vi "InitializeFunctionList.vi"(8 "错误输入（无错误）":errorcluster, 9 "模块定义":T1, 10 "rModuleName":refnum<vi>, 11 "rFunctionList":refnum<vi>) -> (0 "错误输出":errorcluster)   [LabVIEW 2018, in "ModuleInterface.lvlib"]
uses:
  ModuleInterface.lvlib
  ModuleDefinition.ctl
  FunctionItem.ctl
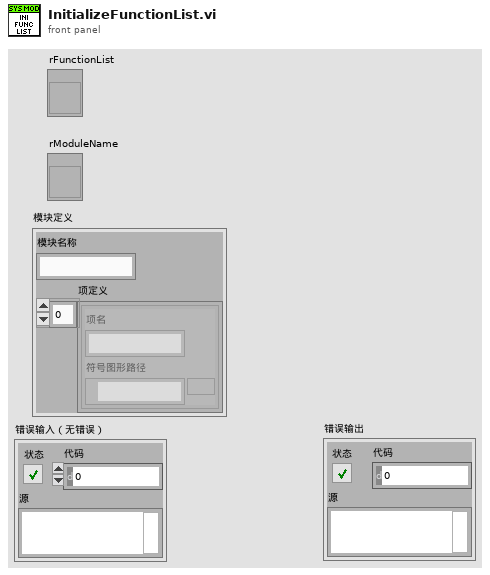
[diagram p1: front panel]
types:
  T1 = typedef "ModuleInterface.lvlib/ModuleDefinition.ctl" = cluster{"模块名称":string, "项定义":T2[]}
  T2 = typedef "ModuleInterface.lvlib/FunctionItem.ctl" = cluster{"项名":string, "符号图形路径":path}
  T3 = typedef "imagedata.ctl" = cluster{"image type":i32, "image depth":i32, "image":u8[], "mask":u8[], "colors":u32[], "Rectangle":cluster{"left":i16, "top":i16, "right":i16, "bottom":i16}}
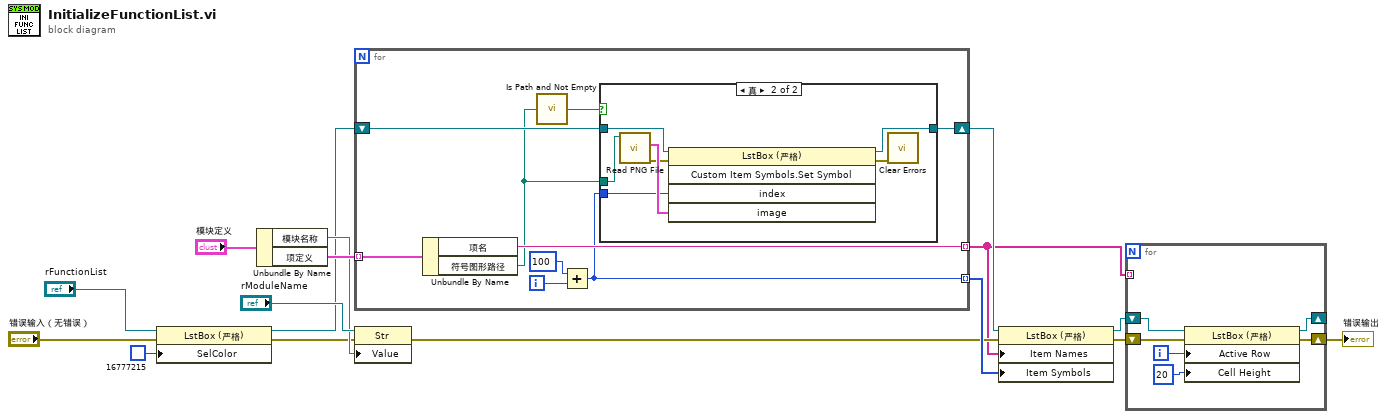
[diagram p0: block diagram]
diagram:
  n1 = property class="LstBox (严格)"(reference="rFunctionList", error in="错误输入（无错误）", "SelColor"=u32 16777215 ("选择颜色")) -> (reference out=w8:refnum<vi>, error out=w6:errorcluster)
  n2 = Unbundle By Name("模块定义") -> ("模块名称"=w10:string, "项定义"=w12:T2[])
  n3 = for {
    tunnel: w12 -> [w25] mode=indexing
    tunnel: [w24] -> w3 mode=indexing
    tunnel: [w20] -> w14 mode=indexing
    shift-right: [w19] -> w15
    shift-left: w8 -> [w21]
    i -> [w22]
    n4 = Unbundle By Name(w25) -> ("项名"=w24:string, "符号图形路径"=w18:path)
    n5 = call <vilib>:"Is Path and Not Empty.vi"("path"=w18) -> ("Is Path and Not Empty?"=w17:bool)  [unwired: 4 in]
    n6 = Add(x=100, y=w22) -> (x+y=w20:i32)
    n7 = case shown="真" w17 {
      tunnel: w21 -> [w26 w33]
      tunnel: w18 -> [_ w32]
      tunnel: w20 -> [_ w29]
      tunnel: [w26 w28] -> w19
      frame False {
      }
      frame True {
        n8 = call <vilib>:"Read PNG File.vi"("path to PNG file"=w32) -> ("error out"=w30:errorcluster, "image data"=w31:T3)  [unwired: 8 in, 1 out]
        n9 = invoke class="LstBox (严格)" method="Custom Item Symbols.Set Symbol"(reference=w33, error in=w30, "index"=w29, "image"=w31) -> (reference out=w28:refnum<vi>, error out=w27:errorcluster)  [unwired: 1 in, 3 out]
        n10 = call <vilib>:"Clear Errors.vi"("error in (no error)"=w27) -> ()  [unwired: 5 in, 2 out]
      }
    }
  }
  n11 = property class="Str"(reference="rModuleName", error in=w6, "Value"=w10) -> (error out=w9:errorcluster)  [unwired: 1 out]
  n12 = property class="LstBox (严格)"(reference=w15, error in=w9, "Item Names"=w3, "Item Symbols"=w14) -> (reference out=w4:refnum<vi>, error out=w2:errorcluster)
  n13 = for {
    tunnel: w3 -> [_] mode=indexing
    shift-right: [w36] -> _
    shift-left: w4 -> [w39]
    shift-right: [w34] -> w1
    shift-left: w2 -> [w35]
    i -> [w38]
    n14 = property class="LstBox (严格)"(reference=w39, error in=w35, "Active Row"=w38, "Cell Height"=20 ("活动行:单元格高度")) -> (reference out=w36:refnum<vi>, error out=w34:errorcluster)
  }
  "错误输出" <- w1
